vi "Error Test.vi"() -> ()   [LabVIEW 2011]
uses:
  JSON GetSet.lvlib
  JSON Value/JSON Value.lvclass
  JSON Scalar/Get as DBL.vi
  JSON Scalar/JSON Scalar.lvclass
  JSON Scalar/Get as Timestamp.vi
  JSON Scalar/Get as EXT.vi
panel:
  in  "JSON stream":string="{\"Value\":123,\"InvlalidValue\":xyz,\"Array\":[1,2,3],\"Time Stamp\": \"2012-10-26 13:28:16.312\",\"Object\":{\"Value\":123,\"Array\":[1,2,3],\"Object\":{\"AAA\":123}}}"
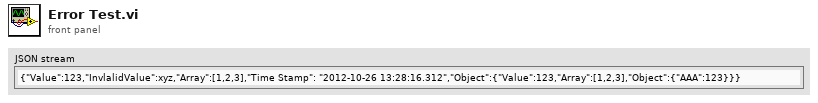
[diagram p1: front panel]
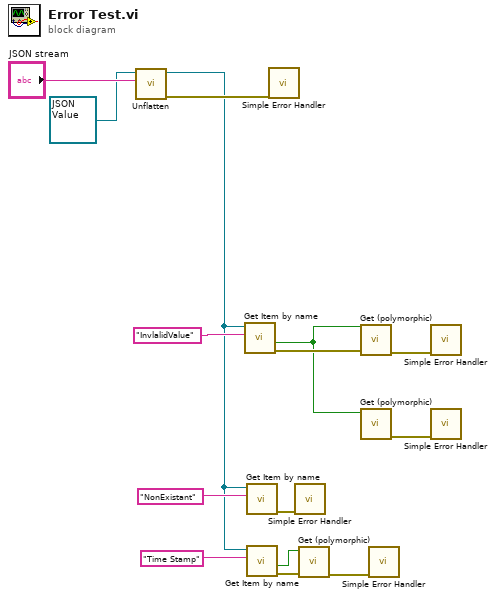
[diagram p0: block diagram]
diagram:
  n1 = call-dynamic "Unflatten.vi"("JSON stream"="JSON stream", "JSON Value in"=refnum<class "JSON Value.lvclass"> refnum) -> ("error out"=w11:errorcluster, "JSON Value out"=w5:refnum<class "JSON Value.lvclass">)  [unwired: 6 in, 2 out]
  n2 = call-dynamic "Get Item by name.vi"("name"="InvlalidValue", "JSON Value In"=w5) -> ("error out"=w10:errorcluster, "found"=w2:bool)  [unwired: 6 in, 2 out]
  n3 = call-dynamic "Get Item by name.vi"("name"="NonExistant", "JSON Value In"=w5) -> ("error out"=w7:errorcluster)  [unwired: 6 in, 3 out]
  n4 = call-dynamic "Get Item by name.vi"("name"="Time Stamp", "JSON Value In"=w5) -> ("error out"=w3:errorcluster, "found"=w1:bool)  [unwired: 6 in, 2 out]
  n5 = call <vilib>:"Simple Error Handler.vi"("error in (no error)"=w11) -> ()  [unwired: 4 in, 5 out]
  n6 = call <vilib>:"Simple Error Handler.vi"("error in (no error)"=w7) -> ()  [unwired: 4 in, 5 out]
  n7 = call-poly "Get (polymorphic).vi"("error in (no error)"=w3, "JSON Value in"=w1) -> ("error out"=w4:errorcluster)  [unwired: 7 in, 2 out]
  n8 = call-poly "Get (polymorphic).vi"("error in (no error)"=w10, "JSON Value in"=w2) -> ("error out"=w15:errorcluster)  [unwired: 7 in, 2 out]
  n9 = call-poly "Get (polymorphic).vi"("JSON Value in"=w2) -> ("error out"=w9:errorcluster)  [unwired: 8 in, 2 out]
  n10 = call <vilib>:"Simple Error Handler.vi"("error in (no error)"=w4) -> ()  [unwired: 4 in, 5 out]
  n11 = call <vilib>:"Simple Error Handler.vi"("error in (no error)"=w15) -> ()  [unwired: 4 in, 5 out]
  n12 = call <vilib>:"Simple Error Handler.vi"("error in (no error)"=w9) -> ()  [unwired: 4 in, 5 out]
